vi "set_template_file.vi"(8 "error in (no error)":errorcluster, 10 "Path":path, 11 "Boc6 in":refnum<class "Boc6.lvclass">) -> (0 "error out":errorcluster, 3 "Boc6 out":refnum<class "Boc6.lvclass">)   [LabVIEW 2017, in "Boc6.lvclass"]
uses:
  Boc6.lvclass
  Report.lvclass
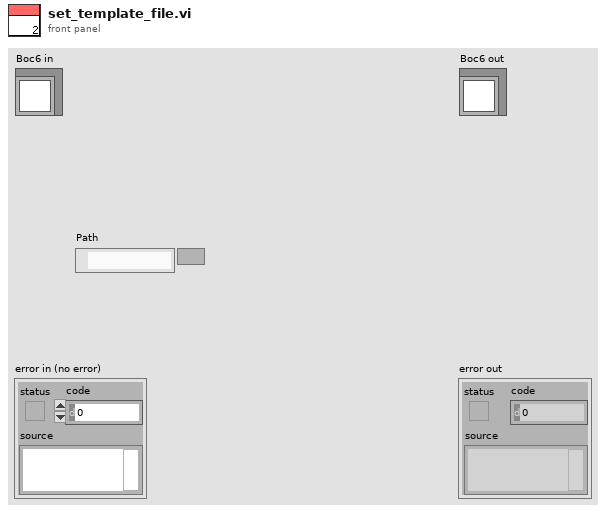
[diagram p1: front panel]
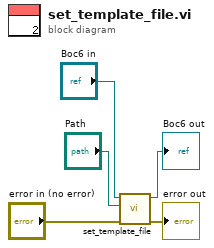
[diagram p0: block diagram]
diagram:
  n1 = call-parent "set_template_file.vi"("error in (no error)"="error in (no error)", "Path"="Path", "Report in"="Boc6 in") -> ("error out"=→"error out":errorcluster, "Report out"=→"Boc6 out":refnum<class "Boc6.lvclass">)  [unwired: 7 in]
